vi "OAT DC Gap Estimator (N Channels).vi"(0 "even-angle signals":cluster{"r0":dbl, "dr":dbl, "Y":dbl[]}[](array[cluster]) {"r0" format="%.2p"; "dr" format="%.2p"; "Y" format="%.2f"}, 1 "even-angle channel info":T2[](array[typedef]) {"channel info"."pregain" format="%.2f"; "channel info"."weighting filter" items=["Linear", "A-weighting", "B-weighting", "C-weighting", "ITU-R 468-4", "Dolby", "CCITT", "C-message", "Wb", "Wc", "Wd", "We", "Wf", "Wh", "Wj", "Wk", "Wm", "AES17 20 kHz lowpass", "AES17 40 kHz lowpass", "AES17 20 kHz highpass", "AES17 40 kHz highpass"]; "channel info"."dB reference" format="%^.1e"; "channel info"."engineering units" items=["custom..."=0, "V"=1, "A"=21, "C"=30, "pC"=31, "s"=32, "-"=29, "Pa"=2, "N"=20, "g"=3, "m/s^2"=4, "m/s"=5, "m"=6, "mm/s"=12, "mm"=13, "micron/s"=14, "micron"=15, "in/s^2"=7, "in/s"=8, "in"=9, "mil/s"=10, "mil"=11, "rad/s^2"=16, "rad/s"=17, "rad"=18, "deg/s^2"=26, "deg/s"=27, "deg"=28, "RPM"=22, "cycle/s^2"=23, "Hz"=24, "cycle"=25, "strain"=19]; "channel info"."sensor sensitivity" format="%#_5f"}, 2 "even-angle position info":T1, 3 "speed profile":T9 {"speed [RPM]" format="%.2f"; "time [s]" format="%.2f"}, 4 "gap references [V]":dbl[](array[numeric]), 5 "error in (no error)":errorcluster, 6 "x-axis selection":u16(ring)=2 items=["Time", "Revolution", "RPM"], 7 "averaging type":enum16{"Linear", "Exponential"}(ring), 8 "reset? (F)":bool, 9 "window":T6(ring), 10 "DC gap unit":u16(ring) items=["V", "EU"]) -> (14 "DC gaps":T8(array[cluster]) {"DC gap value" format="%.2f"; "time/rev/rpm" format="%.2f"}, 15 "unit labels":T7(array[cluster]), 16 "gap position info":T1, 18 "actual gap ref [V]":dbl[](array[numeric]) format="%.2f", 19 "error out":errorcluster)   [LabVIEW 2017, in "SoundVib_RefDataProcess.lvlib"]
doc: "Subtracts the gap reference from the averaged DC gap voltage of the <B>even-angle signal</B> and returns the DC gap in the selected units. The DC gap is a measurement of the movement of the shaft from the reference position to the current position. If <B>gap reference [V]</B> is unwired, the VI computes the <B>actual gap ref [V]</B> from the input signal. Wire data to the <B>even-angle signal</B> input to determine the polymorphic instance to use or manually select the instance."
uses:
  <vilib>/addons/Sound and Vibration/Order Analysis/Referece Data Processing/SoundVib_RefDataProcess.lvlib
  <vilib>/addons/Sound and Vibration/Order Analysis/Tach Process/SubVIs/speed profile.ctl
  <vilib>/addons/Sound and Vibration/Order Analysis/Misc/OAT Position Info.ctl
  <vilib>/addons/_NISVFA/_Shared subVIs/Controls/svc_Resampled Channel Info.ctl
  <vilib>/addons/_NISVFA/_Shared subVIs/Controls/svc_Channel Info.ctl
  <vilib>/addons/_NISVFA/_Shared subVIs/Controls/svc_Engineering Units Text Ring.ctl
  <vilib>/addons/_NISVFA/_Shared subVIs/Controls/svc_Weighting Filter Text Ring.ctl
  <vilib>/addons/Sound and Vibration/Order Analysis/Resample Order Tracking/SoundVib_Resampling.lvlib
  <vilib>/addons/Sound and Vibration/Order Analysis/Tach Process/SoundVib_TachProcess.lvlib
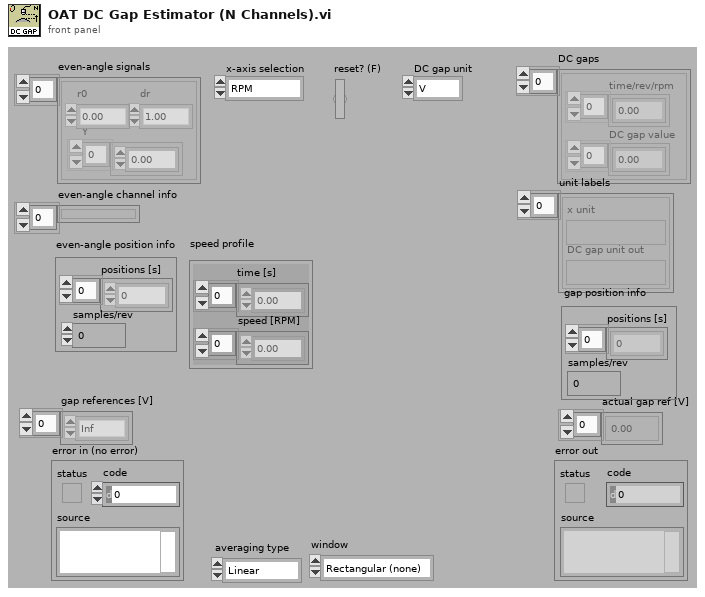
[diagram p1: front panel]
types:
  T1 = typedef "OAT Position Info.ctl" = cluster{"positions [s]":dbl[], "samples/rev":dbl}
  T2 = typedef "svc_Resampled Channel Info.ctl" = cluster{"channel name":string, "description":string, " channel info":T3}
  T3 = typedef "svc_Channel Info.ctl" = cluster{"sensor sensitivity":dbl, "engineering units":T4, "dB reference":dbl, "custom label":string, "weighting filter":T5, "pregain":dbl}
  T4 = typedef "svc_Engineering Units Text Ring.ctl" = u16
  T5 = typedef "svc_Weighting Filter Text Ring.ctl" = u16
  T6 = enum16{"Rectangular (none)", "Hanning", "Low side lobe"}
  T7 = cluster{"x unit":string, "DC gap unit out":string}[]
  T8 = cluster{"time/rev/rpm":dbl[], "DC gap value":dbl[]}[]
  T9 = typedef "SoundVib_TachProcess.lvlib/speed profile.ctl" = cluster{"time [s]":dbl[], "speed [RPM]":dbl[]}
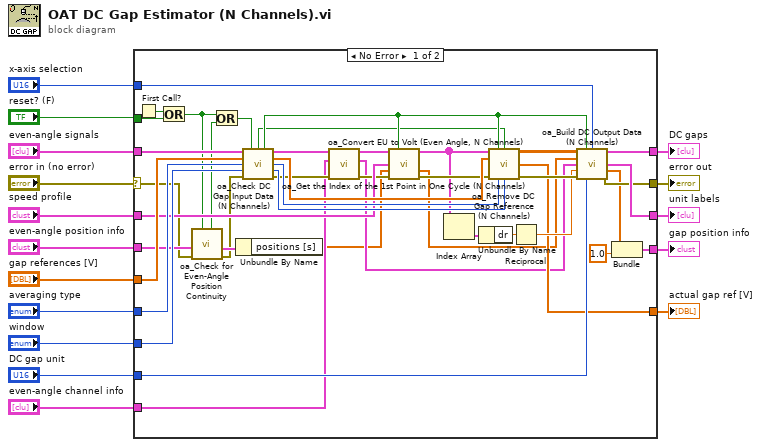
[diagram p0: block diagram]
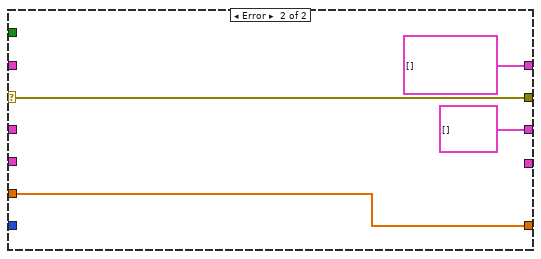
[diagram p2: hidden frame]
diagram:
  n1 = case shown="No Error" "error in (no error)" {
    selector: "error in (no error)" -> [w21 w63]
    tunnel: [w54 w63] -> w15
    tunnel: "even-angle signals" -> [w52 _]
    tunnel: "averaging type" -> [w50 _]
    tunnel: "window" -> [w49 _]
    tunnel: "gap references [V]" -> [w51 w60]
    tunnel: "speed profile" -> [w44 _]
    tunnel: "even-angle position info" -> [w23 _]
    tunnel: "reset? (F)" -> [w28 _]
    tunnel: "x-axis selection" -> [w57 _]
    tunnel: [w56 cluster{"X":dbl[], "Y":dbl[]}[] [] ("DC gaps")] -> w11
    tunnel: [w55 cluster{"X unit":string, "gap unit":string}[] [] ("unit labels")] -> w10
    tunnel: "DC gap unit" -> [w53 _]
    tunnel: [w36 w60] -> w8
    tunnel: [w37 _] -> w7
    tunnel: "even-angle channel info" -> [w30 _]
    frame No Error {
      n2 = First Call?() -> (First Call?: T/F=w29:bool)
      n3 = Or(x=w29, y=w28) -> (x .or. y?=w19:bool)
      n4 = call <vilib>:"oa_Check for Even-Angle Position Continuity.vi"("reset in"=w19, "error in (no error)"=w21, "even-angle position info"=w23) -> ("error out"=w20:errorcluster, "even-angle position info dup"=w22:T1, "position not continuous"=w18:bool)  [unwired: 6 in]
      n5 = Or(x=w19, y=w18) -> (x .or. y?=w17:bool)
      n6 = Unbundle By Name(w22) -> ("positions [s]"=w25:dbl[])
      n7 = call <vilib>:"oa_Check DC Gap Input Data (N Channels).vi"("even angle signals"=w52, "reset?"=w17, "DC gap references [V]"=w51, "averaging type in"=w50, "window in"=w49, "error in (no error)"=w20) -> ("reset DC ref?"=w26:bool, "reset out?"=w27:bool, "even angle signals"=w34:cluster{"r0":dbl, "dr":dbl, "Y":dbl[]}[], "DC gap reference [V]"=w48:dbl[], "averaging type"=w47:enum16{"Linear", "Exponential"}, "window"=w46:T6, "error out"=w35:errorcluster)  [unwired: 3 in]
      n8 = call <vilib>:"oa_Convert EU to Volt (Even Angle, N Channels).vi"("error in (no error)"=w35, "even angle channel info"=w30, "even angle signals"=w34) -> ("error out"=w32:errorcluster, "channel info"=w31:T3[], "even angle signals"=w33:cluster{"r0":dbl, "dr":dbl, "Y":dbl[]}[])  [unwired: 6 in]
      n9 = call <vilib>:"oa_Get the Index of the 1st Point in One Cycle (N Channels).vi"("resampled signal"=w33, "reset? (True)"=w27, "speed profile"=w44, "interpolated pulse positions"=w25, "error in (no error)"=w32) -> ("resampled signal out"=w43:cluster{"r0":dbl, "dr":dbl, "Y":dbl[]}[], "interpolated pulse positions out"=w24:dbl[], "error out"=w45:errorcluster)  [unwired: 8 in]
      n10 = Index Array(array=w43) -> (element=w42:cluster{"r0":dbl, "dr":dbl, "Y":dbl[]})  [unwired: 1 in]
      n11 = Unbundle By Name(w42) -> ("dr"=w41:dbl)
      n12 = call <vilib>:"oa_Remove DC Gap Reference (N Channels).vi"("resampled signal"=w43, "reset?"=w27, "DC ref changed?"=w26, "DC gap reference [V]"=w48, "error in"=w45, "averaging type"=w47, "window"=w46) -> ("DC value out"=w58:dbl[][], "actual gap ref"=w36:dbl[], "error out"=w59:errorcluster)  [unwired: 6 in]
      n13 = Reciprocal(x=w41) -> (1/x=w40:dbl)
      n14 = call <vilib>:"oa_Build DC Output Data (N Channels).vi"("DC value out"=w58, "reset? (True)"=w27, "X axis selection"=w57, "start points"=w24, "channel info"=w31, "samples/rev"=w40, "error in (no error)"=w59, "DC gap unit"=w53) -> ("DC gaps"=w56:cluster{"X":dbl[], "Y":dbl[]}[], "unit labels"=w55:cluster{"X unit":string, "gap unit":string}[], "pulse positions"=w39:dbl[], "error out"=w54:errorcluster)  [unwired: 4 in]
      n15 = Bundle("pulse positions"=w39, 1.0) -> (w37:cluster{"pulse positions":dbl[], dbl})  [unwired: 1 in]
    }
    frame Error {
    }
  }
  "error out" <- w15
  "DC gaps" <- w11
  "unit labels" <- w10
  "actual gap ref [V]" <- w8
  "gap position info" <- w7
